vi "Ev Pic Path.vi"(8 "error in (no error)":errorcluster, 11 "Pic Json Generator in":refnum<class "Pic Json Generator.lvclass">) -> (0 "error out":errorcluster, 3 "Pic Json Generator out":refnum<class "Pic Json Generator.lvclass">)   [LabVIEW 2018, in "Pic Json Generator.lvlib" / "Pic Json Generator.lvclass"]
uses:
  Pic Json Generator.lvclass
  Pic Json Generator.lvclass/Pic Json Generator.ctl
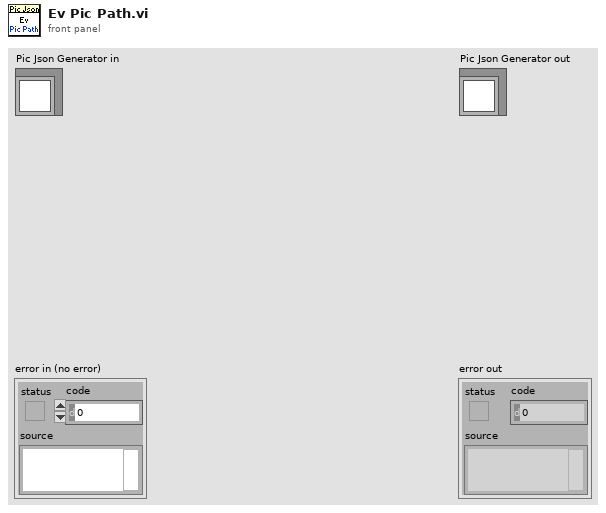
[diagram p1: front panel]
types:
  T1 = typedef "imagedata.ctl" = cluster{"image type":i32, "image depth":i32, "image":u8[], "mask":u8[], "colors":u32[], "Rectangle":cluster{"left":i16, "top":i16, "right":i16, "bottom":i16}}
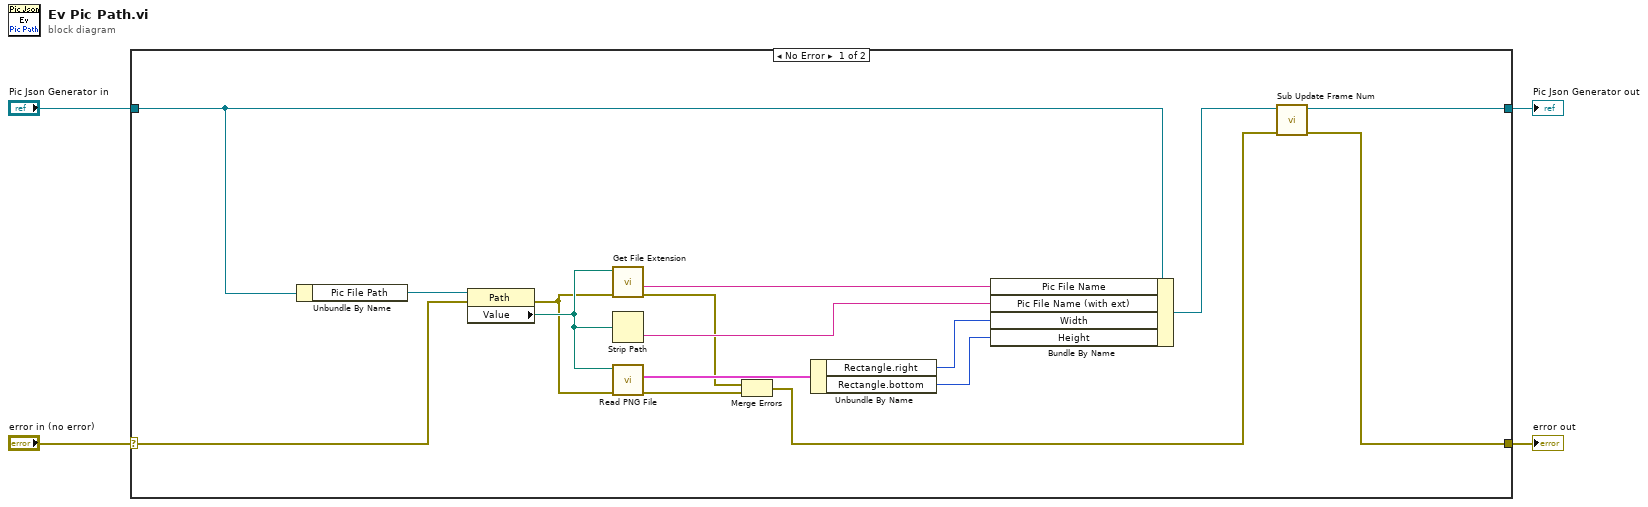
[diagram p0: block diagram]
diagram:
  n1 = case shown="No Error" "error in (no error)" {
    selector: "error in (no error)" -> [w12 w22]
    tunnel: [w5 w22] -> w3
    tunnel: [w6 w21] -> w1
    tunnel: "Pic Json Generator in" -> [w20 w21]
    frame No Error {
      n2 = Unbundle By Name(w20) -> ("Pic File Path"=w19:refnum<vi>)
      n3 = property class="Path"(reference=w19, error in=w12) -> (error out=w11:errorcluster, "Value"=w17:path)  [unwired: 1 out]
      n4 = call <vilib>:"Get File Extension.vi"("error in (no error)"=w11, "file"=w17) -> ("error out"=w9:errorcluster, "filename without extension"=w16:string)  [unwired: 5 in, 3 out]
      n5 = Strip Path(path=w17) -> (name=w15:string)  [unwired: 1 out]
      n6 = call <vilib>:"Read PNG File.vi"("error in (no error)"=w11, "path to PNG file"=w17) -> ("error out"=w10:errorcluster, "image data"=w18:T1)  [unwired: 7 in, 1 out]
      n7 = Merge Errors(w9, w10) -> (w7:errorcluster)
      n8 = Unbundle By Name(w18) -> ("Rectangle.right"=w14:i16, "Rectangle.bottom"=w13:i16)
      n9 = Bundle By Name(cluster=w20, "Pic File Name"=w16, "Pic File Name (with ext)"=w15, "Width"=w14, "Height"=w13) -> (w8:refnum<class "Pic Json Generator.lvclass">)
      n10 = call "Sub Update Frame Num.vi"("error in (no error)"=w7, "Pic Json Generator in"=w8) -> ("error out"=w5:errorcluster, "Pic Json Generator out"=w6:refnum<class "Pic Json Generator.lvclass">)  [unwired: 8 in]
    }
    frame Error {
    }
  }
  "error out" <- w3
  "Pic Json Generator out" <- w1
